vi "Test Logging Directory.vi"() -> (3 "test logging directory":path)   [LabVIEW 2018]
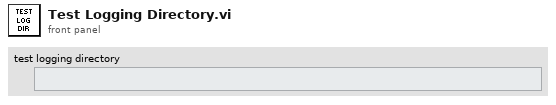
[diagram p1: front panel]
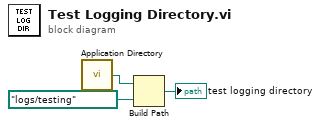
[diagram p0: block diagram]
diagram:
  n1 = call <vilib>:"Application Directory.vi"() -> ("Application Directory"=w1:path)
  n2 = Build Path(base path=w1, name or relative path=path "logs/testing") -> (appended path=→"test logging directory":path)
